vi "Set_Pin_Status.vi"(6 "Valor pin":string(combo), 8 "error in (no error)":errorcluster, 9 "PIN":i32, 10 "CH":i32, 11 "NXP in":refnum<class "NXP.lvclass">) -> (0 "error out":errorcluster, 1 "Expected Response":string, 2 "Command to Send":string, 3 "NXP out":refnum<class "NXP.lvclass">)   [LabVIEW 2020, in "NXP.lvclass"]
uses:
  NXP.lvclass
  Abstract/Serial Device/Serial Device.lvclass
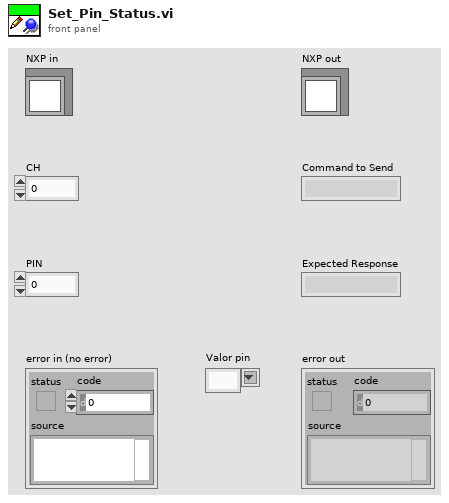
[diagram p1: front panel]
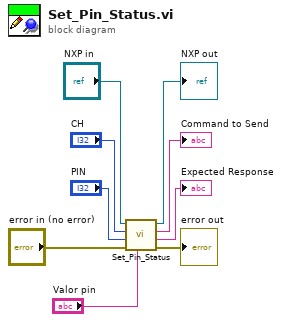
[diagram p0: block diagram]
diagram:
  n1 = call-parent "Set_Pin_Status.vi"("Valor pin"="Valor pin", "error in (no error)"="error in (no error)", "PIN"="PIN", "CH"="CH", "Serial Device in"="NXP in") -> ("error out"=→"error out":errorcluster, "Expected Response"=→"Expected Response":string, "Command to Send"=→"Command to Send":string, "Serial Device out"=→"NXP out":refnum<class "NXP.lvclass">)  [unwired: 3 in]
